vi "Path or Name.vi"(11 "Full Path (with $) or Name":string) -> (3 "Relative Path or JSON-format name":string)   [LabVIEW 2017, in "JSONtext.lvlib"]
uses:
  JSONtext.lvlib
  support/quote and escape json string 2.vi
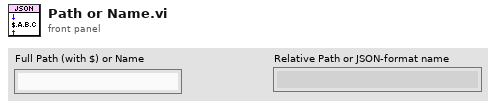
[diagram p1: front panel]
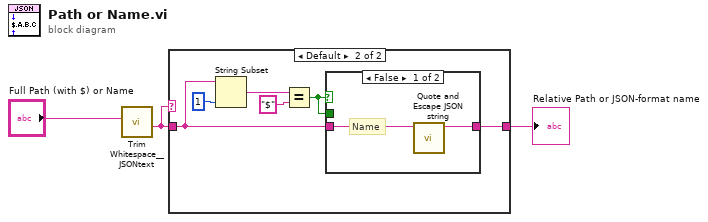
[diagram p0: block diagram]
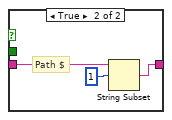
[diagram p3: hidden frame]
diagram:
  n1 = call "Trim Whitespace__JSONtext.vi"("String in"="Full Path (with $) or Name") -> ("String out"=w1:string)  [unwired: 6 in]
  n2 = case shown="Default" w1 {
    tunnel: w1 -> [_ w5]
    tunnel: [_ w4] -> w2
    frame "" {
    }
    frame Default {
      n3 = String Subset(string=w5, length (rest)=1 ("length (rest)")) -> (substring=w9:string)  [unwired: 1 in]
      n4 = Equal?(x=w9, y="$") -> (x = y?=w6:bool)
      n5 = case shown="False" w6 {
        tunnel: w6 -> [_ _]
        tunnel: w5 -> [w11 w14]
        tunnel: [w10 w12] -> w4
        frame False {
          # "Name"
          n6 = call "Quote and Escape JSON string.vi"("Plain Text"=w11) -> ("<JSON>"=w10:string)  [unwired: 10 in]
        }
        frame True {
          # "Path $"
          n7 = String Subset(string=w14, offset (0)=1) -> (substring=w12:string)  [unwired: 1 in]
        }
      }
    }
  }
  "Relative Path or JSON-format name" <- w2
